vi "Test Factory.vi"() -> ()   [LabVIEW 2013]
uses:
  Control Packets/ControlPacket/ControlPacket.lvclass
panel:
  out "Array":refnum<class "ControlPacket.lvclass">[](array[class])
  out "Remaining Packets":u8[](array[numeric]) format="%08b"
  in  "stop":bool
  out "error out":errorcluster
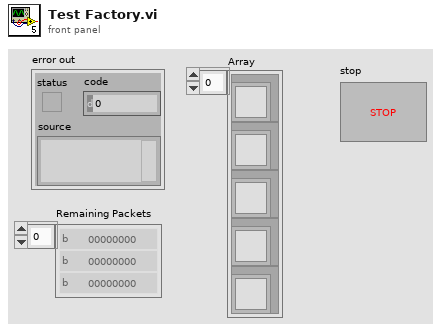
[diagram p1: front panel]
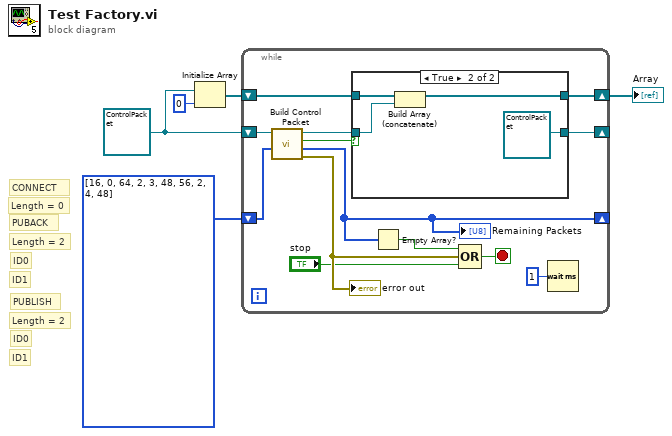
[diagram p0: block diagram]
diagram:
  w3 = refnum<class "ControlPacket.lvclass"> refnum ("ControlPacket.lvclass")
  # "ID1"
  # "ID0"
  # "Length = 2"
  # "PUBLISH"
  # "ID1"
  # "ID0"
  # "Length = 2"
  # "PUBACK"
  # "Length = 0"
  # "CONNECT"
  n1 = Initialize Array(w3, 0 ("dimension size")) -> (w4:refnum<class "ControlPacket.lvclass">[])
  n2 = while {
    shift-right: [w15] -> _
    shift-left: w3 -> [w17]
    shift-right: [w6] -> _
    shift-left: u8[] [16, 0, 64, 2, 3, 48, 56, 2, 4, 48] ("Incoming Packets") -> [w18]
    shift-right: [w7] -> w1
    shift-left: w4 -> [w9]
    stop <- w12 stop-if-true
    n3 = call "Build Control Packet.vi"("Incoming Packets"=w18, "Incomplete ControlPacket"=w17) -> ("error out"=w13:errorcluster, "Remaining Packets"=w6:u8[], "Complete Packet"=w16:bool, "ControlPacket"=w14:refnum<class "ControlPacket.lvclass">)  [unwired: 6 in]
    "error out" <- w13
    "Remaining Packets" <- w6
    n4 = case shown="True" w16 {
      tunnel: [w20 refnum<class "ControlPacket.lvclass"> refnum ("ControlPacket.lvclass")] -> w15
      tunnel: w14 -> [w20 w22]
      tunnel: w9 -> [w19 w23]
      tunnel: [w19 w21] -> w7
      frame False {
      }
      frame True {
        n5 = Build Array (concatenate)(w23, w22) -> (w21:refnum<class "ControlPacket.lvclass">[])
      }
    }
    n6 = Empty Array?(array=w6) -> (empty?=w8:bool)
    n7 = Compound Arithmetic op=OR(w8, w13, "stop") -> (w12:bool)
    n8 = Wait (ms)(milliseconds to wait=u32 1) -> ()  [unwired: 1 out]
  }
  "Array" <- w1
